vi "Write row.vi"(8 "error in (no error)":errorcluster, 10 "row":u8, 11 "BoardField in":refnum<class "BoardField.lvclass">) -> (0 "error out":errorcluster, 3 "BoardField out":refnum<class "BoardField.lvclass">)   [LabVIEW 2017, in "BoardField.lvclass"]
uses:
  BoardField.lvclass
  BoardField.lvclass/BoardField.ctl
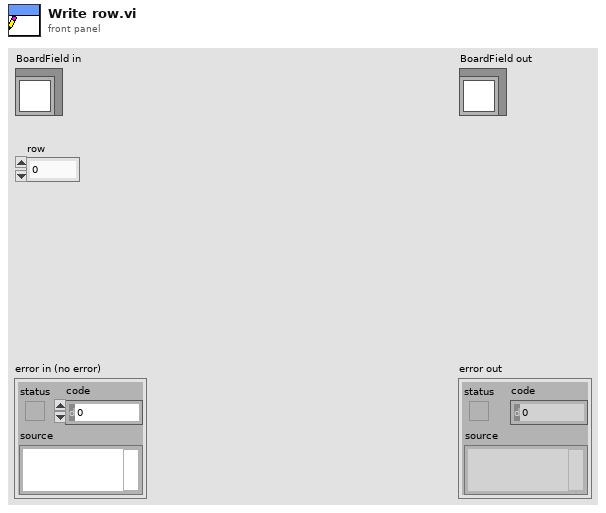
[diagram p1: front panel]
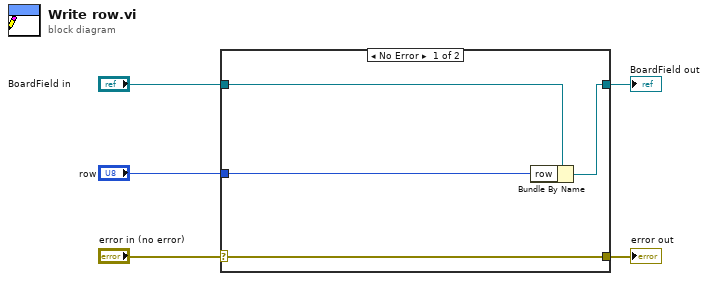
[diagram p0: block diagram]
diagram:
  n1 = case shown="No Error" "error in (no error)" {
    selector: "error in (no error)" -> [w9 w10]
    tunnel: [w9 w10] -> w4
    tunnel: [w7 w11] -> w2
    tunnel: "BoardField in" -> [w8 w11]
    tunnel: "row" -> [w6 _]
    frame No Error {
      n2 = Bundle By Name(cluster=w8, "row"=w6) -> (w7:refnum<class "BoardField.lvclass">)
    }
    frame Error {
    }
  }
  "error out" <- w4
  "BoardField out" <- w2
